vi "find_visa_com_resources.vi"(1 "error in (no error)":errorcluster) -> (2 "Number of COM Resources Found":i32, 3 "Resource Names of All COM Devices Found":string[](array[string]), 4 "error out":errorcluster)   [LabVIEW 2017]
doc: "This VI finds the VISA Resource Names of all COM ports on the host machine. It first finds the VISA Resource Names of all serial ports and then filters through these to find which of those are COM ports."
panel:
  # "Find VISA COM Resource Names:\nThis VI finds the VISA Resource Names of all\nCOM ports on the host machine.  Just run the VI\nto find how many COM ports are found and to\nobtain an array of their VISA Resource Names."
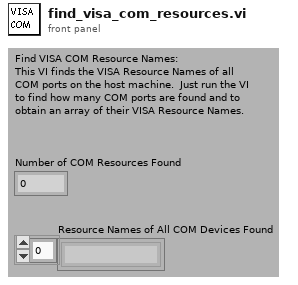
[diagram p1: front panel]
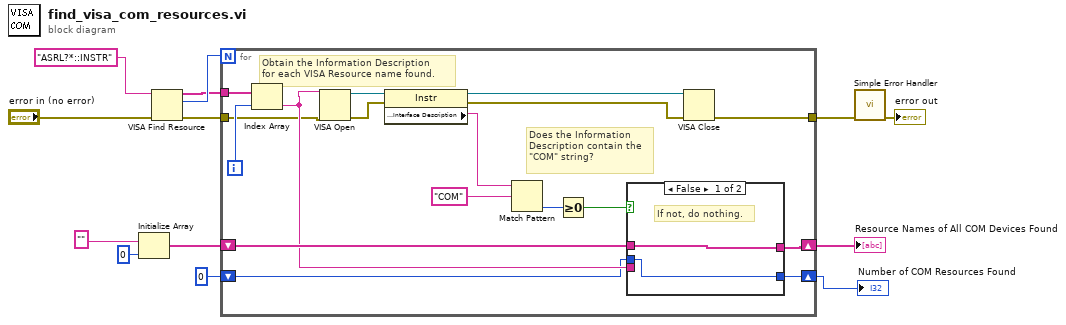
[diagram p0: block diagram]
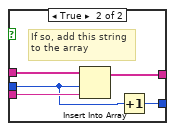
[diagram p2: hidden frame]
diagram:
  n1 = Initialize Array("", 0 ("dimension size")) -> (w8:string[])
  n2 = VISA Find Resource(8:"error in (no error)", 11:"ASRL?*::INSTR" ("expression (\"\")")) -> (0:w6:errorcluster, 2:w12:u32, 3:w11:string[])  [unwired: 1 in]
  n3 = for {
    N: w12 -> [_]
    tunnel: w11 -> [w27]
    shift-right: [w18] -> w7
    shift-left: w8 -> [w21]
    tunnel: w6 -> [w17]
    tunnel: [w16] -> w5
    shift-right: [w14] -> w1
    shift-left: 0 -> [w15]
    i -> [w22]
    # "Obtain the Information Description\nfor each VISA Resource name found."
    # "Does the Information \nDescription contain the\n\"COM\" string?"
    n4 = Index Array(array=w27, index=w22) -> (element=w19:string)
    n5 = VISA Open(error in (no error)=w17, VISA resource name=w19) -> (VISA resource name=w20:refnum<visa-resource-name>, error out=w29:errorcluster)  [unwired: 3 in]
    n6 = property class="Instr"(reference=w20, error in=w29) -> (reference out=w30:refnum<visa-resource-name>, error out=w28:errorcluster, "Interface Information:Interface Description"=w26:string)
    n7 = Match Pattern(string=w26, regular expression="COM") -> (offset past match=w24:i32)  [unwired: 1 in, 3 out]
    n8 = Greater Or Equal To 0?(x=w24) -> (x >= 0?=w23:bool)
    n9 = case shown="False" w23 {
      tunnel: w15 -> [w31 w34]
      tunnel: [w32 w37] -> w18
      tunnel: w21 -> [w32 w36]
      tunnel: w19 -> [_ w35]
      tunnel: [w31 w33] -> w14
      frame False {
        # "If not, do nothing."
      }
      frame True {
        # "If so, add this string\nto the array"
        n10 = Insert Into Array(array=w36, index=w34, new element=w35) -> (w37:string[])
        n11 = Increment(x=w34) -> (x+1=w33:i32)
      }
    }
    n12 = VISA Close(VISA resource name=w30, error in (no error)=w28) -> (error out=w16:errorcluster)
  }
  "Number of COM Resources Found" <- w1
  "Resource Names of All COM Devices Found" <- w7
  n13 = call <vilib>:"Simple Error Handler.vi"("error in (no error)"=w5) -> ("error out"=→"error out":errorcluster)  [unwired: 4 in, 4 out]
